vi "Fixed Time Graph Read.vi"(8 "error in":errorcluster, 9 "Data to read in":T2, 10 "Channel_Timing in":T1, 11 "Report Viewer in":refnum<class "Report Viewer.lvclass">) -> (0 "error out":errorcluster, 1 "Data to read out":T2, 2 "Channel_Timing out":T1, 3 "Report Viewer out":refnum<class "Report Viewer.lvclass">, 4 "Waveform":waveform(dbl))   [LabVIEW 2023, in "Report Viewer.lvlib" / "Report Viewer.lvclass"]
uses:
  Library/Report Viewer.lvclass
  Custom Controls/Channel_Timing.ctl
  Custom Controls/Data to Read.ctl
  Library/Report Viewer.lvclass/Report Viewer.ctl
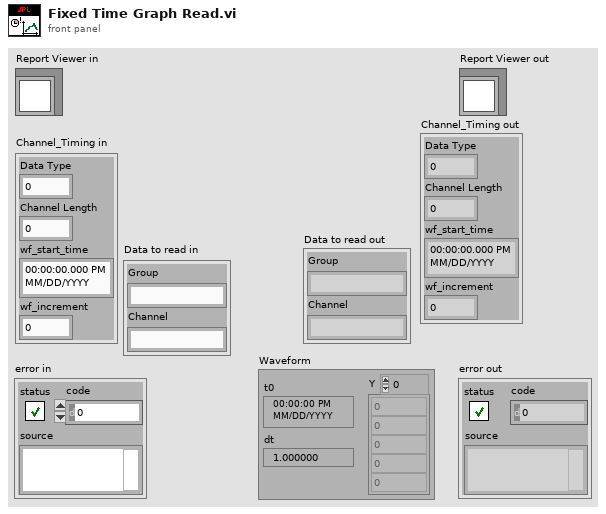
[diagram p1: front panel]
types:
  T1 = typedef "Report Viewer.lvlib/Report Viewer.lvclass/Channel_Timing.ctl" = cluster{"Data Type":u16, "Channel Length":u64, "wf_start_time":timestamp, "wf_increment":dbl}
  T2 = typedef "Report Viewer.lvlib/Report Viewer.lvclass/Data to Read.ctl" = cluster{"Group":string, "Channel":string}
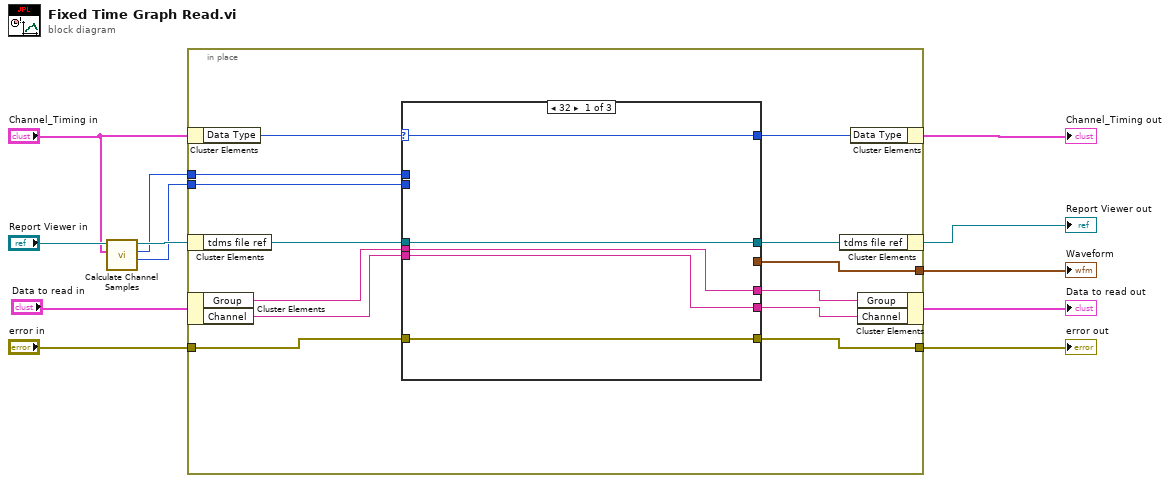
[diagram p0: block diagram]
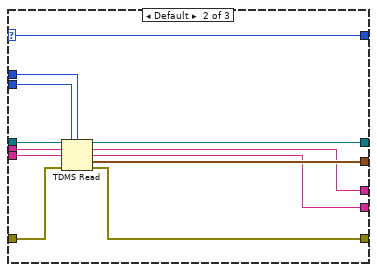
[diagram p2: hidden frame]
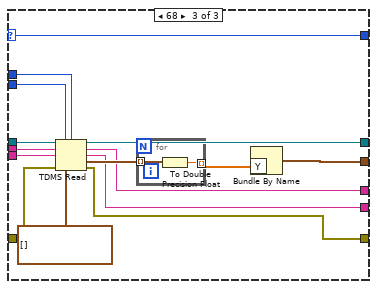
[diagram p3: hidden frame]
diagram:
  n1 = call "Calculate Channel Samples.vi"("Channel Timing"="Channel_Timing in", "Report Viewer in"="Report Viewer in") -> ("Sample Offset"=w1:u32, "Num_Samples"=w2:u32, "Report Viewer out"=w4:refnum<class "Report Viewer.lvclass">)  [unwired: 6 in, 1 out]
  n2 = in-place {
    in-place-border: [w23] -> w11
    in-place-border: "error in" -> [w22]
    in-place-border: [w19] -> w8
    in-place-border: w2 -> [w14]
    in-place-border: w1 -> [w13]
    n3 = in-place-cluster #1("Channel_Timing in") -> ("Data Type"=w21:u16)
    n4 = in-place-cluster #2(w4) -> ("tdms file ref"=w25:refnum<k34>)
    n5 = in-place-cluster #3("Data to read in") -> ("Group"=w18:string, "Channel"=w17:string)
    n6 = case shown="32" w21 {
      selector: w21 -> [w30 w38 w53]
      tunnel: w25 -> [w29 w42 w57]
      tunnel: [w29 w41 w55] -> w24
      tunnel: [w28 w40 w48] -> w23
      tunnel: w22 -> [w28 w39 w56]
      tunnel: w13 -> [_ w35 w52]
      tunnel: w14 -> [_ w36 w51]
      tunnel: [w30 w38 w53] -> w20
      tunnel: [_ w37 w47] -> w19
      tunnel: w18 -> [w27 w34 w46]
      tunnel: w17 -> [w26 w33 w45]
      tunnel: [w27 w32 w44] -> w16
      tunnel: [w26 w31 w43] -> w15
      frame 32 {
      }
      frame Default {
        n7 = TDMS Read(0:w42, 1:w35, 2:w36, 5:w34, 7:w33, 11:w39) -> (4:w41:refnum<k34>, 6:w32:string, 8:w31:string, 10:w37:waveform(dbl), 15:w40:errorcluster)  [unwired: 2 in, 1 out]
      }
      frame 68 {
        n8 = TDMS Read(0:w57, 1:w52, 2:w51, 5:w46, 7:w45, 11:w56, 12:timestamp[] []) -> (4:w55:refnum<k34>, 6:w44:string, 8:w43:string, 10:w49:timestamp[], 15:w48:errorcluster)  [unwired: 1 in, 1 out]
        n9 = for {
          tunnel: w49 -> [w59] mode=indexing
          tunnel: [w58] -> w50 mode=indexing
          n10 = To Double Precision Float(number=w59) -> (double precision float=w58:dbl)
        }
        n11 = Bundle By Name("Y"=w50) -> (w47:waveform(dbl))  [unwired: 1 in]
      }
    }
    n12 = in-place-cluster #2("tdms file ref"=w24) -> (→"Report Viewer out":refnum<class "Report Viewer.lvclass">)
    n13 = in-place-cluster #1("Data Type"=w20) -> (→"Channel_Timing out":T1)
    n14 = in-place-cluster #3("Group"=w16, "Channel"=w15) -> (→"Data to read out":T2)
  }
  "error out" <- w11
  "Waveform" <- w8
